vi "Get Elapsed Time.vi"(8 "error in (no error)":errorcluster, 11 "Elapsed Time.lvclass in":refnum<class "Elapsed Time.lvclass">) -> (0 "error out":errorcluster, 2 "Elapsed Time [s]":dbl, 3 "Elapsed Time.lvclass out":refnum<class "Elapsed Time.lvclass">)   [LabVIEW 2015, in "Elapsed Time.lvclass"]
doc: "Returns the time (in seconds) since the elapsed time was reset."
uses:
  Elapsed Time.lvclass
  Elapsed Time.lvclass/Elapsed Time.ctl
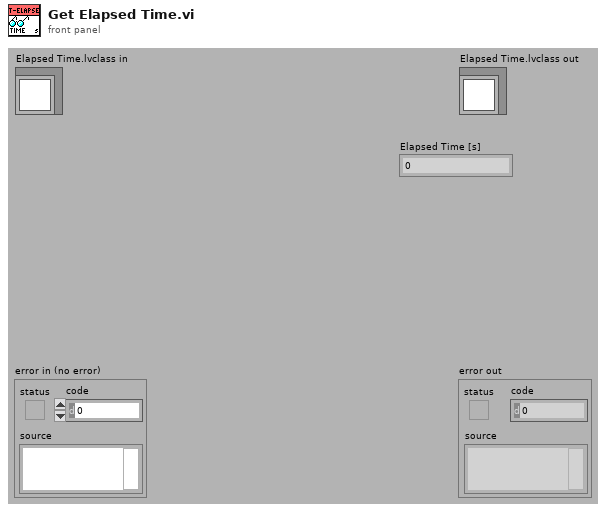
[diagram p1: front panel]
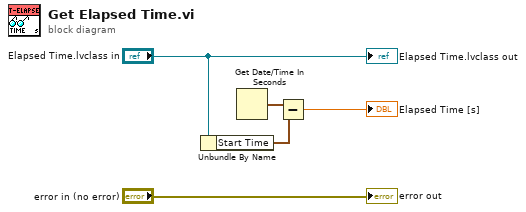
[diagram p0: block diagram]
diagram:
  n1 = Unbundle By Name("Elapsed Time.lvclass in") -> ("Start Time"=w1:timestamp)
  n2 = Get Date/Time In Seconds() -> (seconds since 1Jan1904=w2:timestamp)
  n3 = Subtract(x=w2, y=w1) -> (x-y=→"Elapsed Time [s]":dbl)
  "error out" <- "error in (no error)"
  "Elapsed Time.lvclass out" <- "Elapsed Time.lvclass in"
